vi "Bounce Window_Set Password.vi"() -> (3 "新密碼 Out":string)   [LabVIEW 2015]
uses:
  <vilib>/Utility/miscctls.llb/LVPointTypeDef.ctl
panel:
  in  "登入":bool
  in  "確認 :":string
  in  "新密碼 :":string
  # "密碼設定"
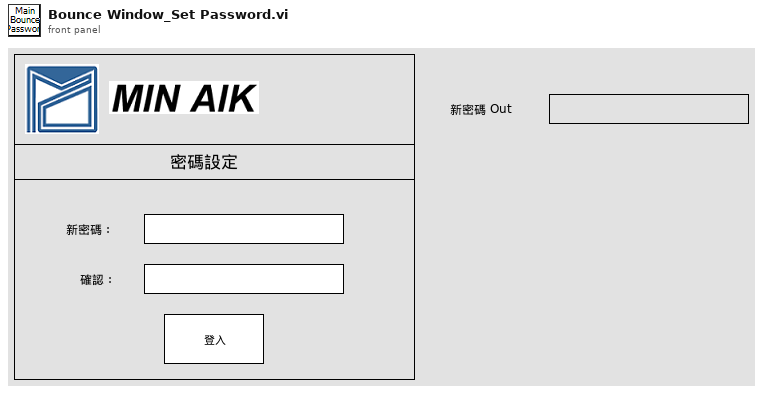
[diagram p1: front panel]
types:
  T1 = typedef "LVPointTypeDef.ctl" = cluster{"Horizontal":i16, "Vertical":i16}
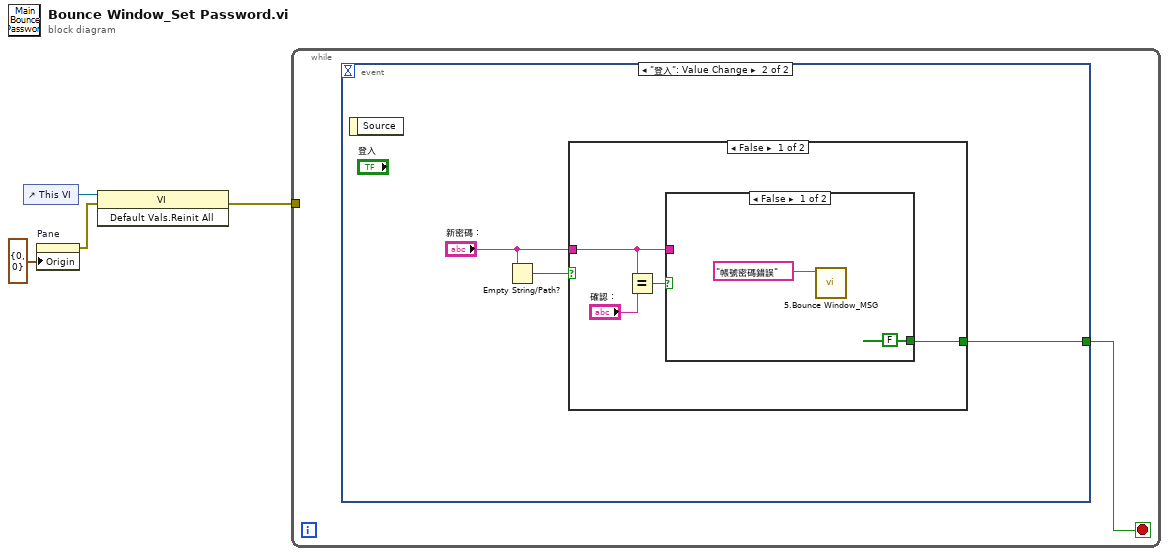
[diagram p0: block diagram]
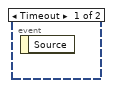
[diagram p2: hidden frame]
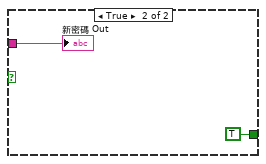
[diagram p3: hidden frame]
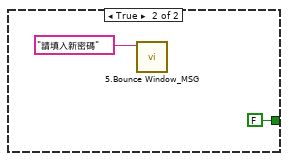
[diagram p4: hidden frame]
diagram:
  n1 = control-ref of="This VI"() -> (w3:refnum<vi>)
  n2 = property on="Pane" class="Pane"("Origin"=T1 {"Horizontal"=0, "Vertical"=0}) -> (error out=w2:errorcluster)  [unwired: 2 in, 1 out]
  n3 = invoke class="VI" method="Default Vals.Reinit All"(reference=w3, error in=w2) -> (error out=w1:errorcluster)  [unwired: 1 in, 2 out]
  n4 = while {
    tunnel: w1 -> [_]
    stop <- w5 stop-if-true
    n5 = event shown="[1] \"登入\": Value Change" {
      selector: _ -> [_ _]
      dyn-events: _ -> [_ _]
      timeout: _ -> [_ _]
      tunnel: [_ w8] -> w5
      event Timeout {
        n6 = event-data() -> ()  [unwired: 1 in, 1 out]
      }
      event "登入": Value Change {
        n7 = event-data() -> ()  [unwired: 1 in, 1 out]
        n8 = Empty String/Path?(string/path="新密碼 :") -> (empty?=w6:bool)
        n9 = case shown="False" w6 {
          tunnel: [w10 FALSE] -> w8
          tunnel: "新密碼 :" -> [w9 _]
          frame False {
            n10 = Equal?(x=w9, y="確認 :") -> (x = y?=w12:bool)
            n11 = case shown="False" w12 {
              tunnel: [FALSE TRUE] -> w10
              tunnel: w9 -> [_ w16]
              frame False {
                n12 = call "5.Bounce Window_MSG.vi"("MSG In"="帳號密碼錯誤" ("message")) -> ()  [unwired: 11 in]
              }
              frame True {
                "新密碼 Out" <- w16
              }
            }
          }
          frame True {
            n13 = call "5.Bounce Window_MSG.vi"("MSG In"="請填入新密碼" ("message")) -> ()  [unwired: 11 in]
          }
        }
      }
    }
  }
